vi "File Rename.vi"(8 "RadioBtnsControl Refnum 2":refnum<vi>, 9 "RadioBtnsControl Refnum":refnum<vi>, 10 "Label.Text":string, 11 "selected path":path) -> (0 "CRC file refnum":refnum<file>, 1 "CRC File Path":path, 2 "refnum out":refnum<file>, 3 "Path":path)   [LabVIEW 2020]
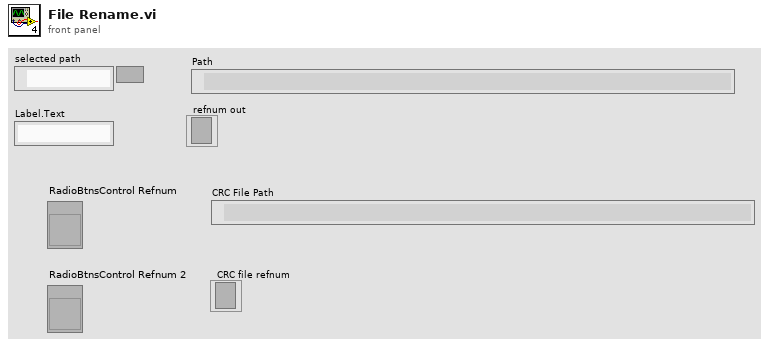
[diagram p1: front panel]
types:
  T1 = enum16{"open", "replace", "create", "open or create", "replace or create", "replace or create with confirmation"}
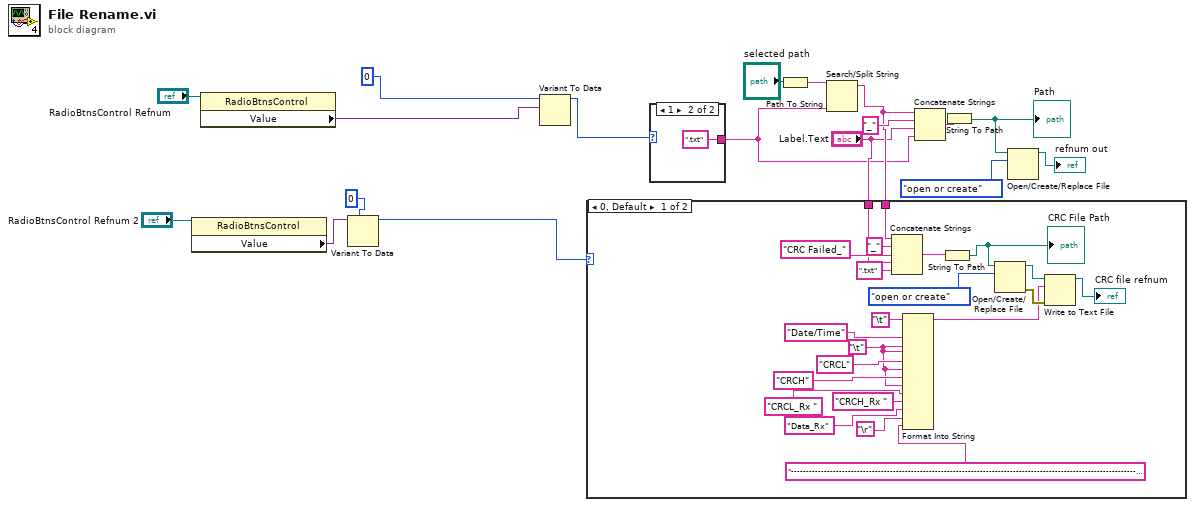
[diagram p0: block diagram]
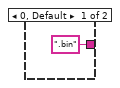
[diagram p3: hidden frame]
diagram:
  n1 = property class="RadioBtnsControl"(reference="RadioBtnsControl Refnum 2") -> ("Value"=w2:variant)  [unwired: 1 in, 2 out]
  n2 = property class="RadioBtnsControl"(reference="RadioBtnsControl Refnum") -> ("Value"=w10:variant)  [unwired: 1 in, 2 out]
  n3 = Variant To Data(type=u32 0, Variant=w2) -> (data=w1:u32)  [unwired: 1 in, 1 out]
  n4 = Variant To Data(type=u32 0, Variant=w10) -> (data=w8:u32)  [unwired: 1 in, 1 out]
  n5 = case shown="1" w8 {
    tunnel: [".bin" ("string") ".txt" ("string")] -> w5
    frame 0, Default {
    }
    frame 1 {
    }
  }
  n6 = Path To String(path="selected path") -> (string=w17:string)
  n7 = Search/Split String(string=w17, search string/char (-)=w5) -> (substring before match=w7:string)  [unwired: 1 in, 2 out]
  n8 = case shown="0, Default" w1 {
    tunnel: w7 -> [w42 _]
    tunnel: "Label.Text" -> [w36 _]
    frame 0, Default {
      w28 = "\t"
      n9 = Concatenate Strings(w42, "_" ("string"), "CRC Failed_" ("string"), w36, ".txt" ("string")) -> (w39:string)
      n10 = Format Into String(initial string="\t", "Date/Time" ("text"), w28, w28, "CRCL" ("input 4"), w28, "CRCH" ("input 6"), w28, "CRCL_Rx " ("input 8"), "CRCH_Rx " ("input 9"), "Data_Rx" ("input 10"), "\r", "------------------------------------------------------------------------------------------------------------------------------------" ("input 13")) -> (resulting string=w24:string)  [unwired: 2 in, 1 out]
      n11 = String To Path(string=w39) -> (path=w38:path)
      "CRC File Path" <- w38
      n12 = Open/Create/Replace File(file path (use dialog)=w38, operation (0:open)=T1."open or create") -> (refnum out=w33:refnum<file>, error out=w34:errorcluster)  [unwired: 4 in, 1 out]
      n13 = Write to Text File(file (use dialog)=w33, text=w24, error in=w34) -> (refnum out=→"CRC file refnum":refnum<file>)  [unwired: 1 in, 2 out]
    }
    frame 1 {
    }
  }
  n14 = Concatenate Strings(w7, "_" ("string"), "Label.Text", w5) -> (w18:string)
  n15 = String To Path(string=w18) -> (path=w14:path)
  "Path" <- w14
  n16 = Open/Create/Replace File(file path (use dialog)=w14, operation (0:open)=T1."open or create") -> (refnum out=→"refnum out":refnum<file>)  [unwired: 4 in, 2 out]
